vi "Write - Async.vi"(8 "error in":errorcluster, 10 "write":string, 11 "Serial IO in":refnum<class "Serial IO.lvclass">) -> (0 "error out":errorcluster, 3 "Serial IO out":refnum<class "Serial IO.lvclass">)   [LabVIEW 2015, in "Serial IO.lvclass"]
uses:
  Serial IO.lvclass
  Serial IO.lvclass/Serial IO.ctl
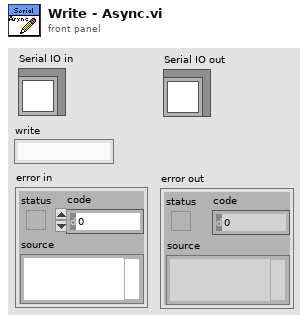
[diagram p1: front panel]
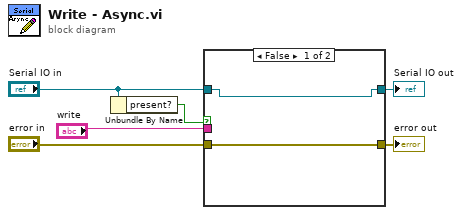
[diagram p0: block diagram]
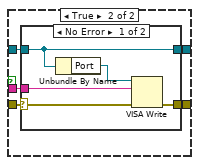
[diagram p2: hidden frame]
diagram:
  n1 = Unbundle By Name("Serial IO in") -> ("present?"=w1:bool)
  n2 = case shown="False" w1 {
    tunnel: "error in" -> [w7 w13]
    tunnel: [w7 w12] -> w5
    tunnel: [w8 w11] -> w4
    tunnel: "write" -> [_ w10]
    tunnel: "Serial IO in" -> [w8 w9]
    frame False {
    }
    frame True {
      n3 = case shown="No Error" w13 {
        selector: w13 -> [w15 w20]
        tunnel: [w14 w20] -> w12
        tunnel: [w18 w19] -> w11
        tunnel: w9 -> [w18 w19]
        tunnel: w10 -> [w16 _]
        frame No Error {
          n4 = Unbundle By Name(w18) -> ("Port"=w17:refnum<visa-resource-name>)
          n5 = VISA Write(VISA resource name=w17, write buffer=w16, error in (no error)=w15) -> (error out=w14:errorcluster)  [unwired: 2 out]
        }
        frame Error {
        }
      }
    }
  }
  "error out" <- w5
  "Serial IO out" <- w4
